vi "EventBuilder.publish event data service.vi"(0 "i ref in":refnum<vi>, 1 "eventID":i32=-1, 2 "eventData":T1, 3 "ms timeout (10000)":i32=10000, 5 "error in (no error)":errorcluster) -> (14 "i ref out":refnum<vi>, 17 "timed out":bool, 19 "error out":errorcluster)   [LabVIEW 2014, in "EventBuilder.lvlib"]
doc: "Publishes the service \"EVENTBUILDERNAME_eventData\".\n\nIf the service does not exist, it will be created. If the service data changes its size, the service is destroyed and recreated."
uses:
  EventBuilder.lvlib
  CS_Core/CSSystem/CoreDefs/CoreDefs.rawDataType.ctl
  CS_Core/CSSystem/CSSystemLib/CSSystemLib.lvlib
  CSlibraries-extern/DimLVEvent/LVDimInterface/LVDimInterface.lvlib
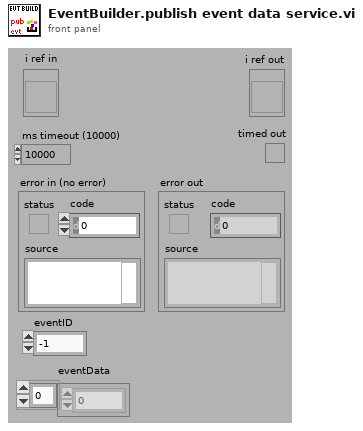
[diagram p1: front panel]
types:
  T1 = typedef "CoreDefs.rawDataType.ctl" = i8[]
  T2 = typedef "EventBuilder.lvlib/EventBuilder.i attribute.ctl" = cluster{"header":string, "DAQObjs":string[], "headerID":dbl, "eventID":i32, "dataDescriptionID":i32, "eventDataID":i32, "eventDataSize":i32, "dataDescriptionSize":i32}
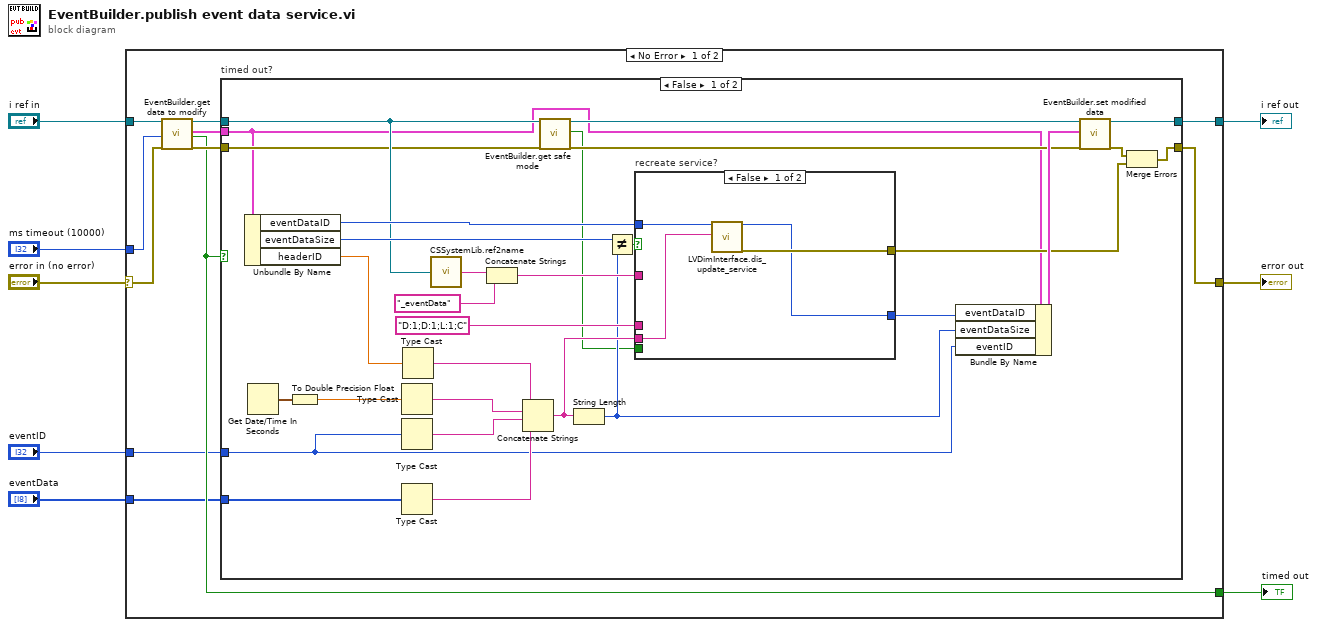
[diagram p0: block diagram]
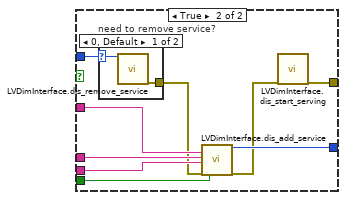
[diagram p2: hidden frame]
diagram:
  n1 = case shown="No Error" "error in (no error)" {
    selector: "error in (no error)" -> [w11 w67]
    tunnel: "i ref in" -> [w19 w68]
    tunnel: [w18 w67] -> w5
    tunnel: [w17 w68] -> w7
    tunnel: "ms timeout (10000)" -> [w13 _]
    tunnel: [w12 _] -> w3
    tunnel: "eventData" -> [w10 _]
    tunnel: "eventID" -> [w9 _]
    frame No Error {
      n2 = call "EventBuilder.get data to modify.vi"("i ref in"=w19, "ms timeout (10000)"=w13, "error in (no error)"=w11) -> ("i ref out"=w16:refnum<vi>, "i attribute"=w14:T2, "timed out"=w12:bool, "error out"=w15:errorcluster)  [unwired: 13 in]
      n3 = case "timed out?" shown="False" w12 {
        tunnel: [w39 w65] -> w18
        tunnel: [w49 w66] -> w17
        tunnel: w16 -> [w25 w66]
        tunnel: w15 -> [w23 w65]
        tunnel: w14 -> [w21 _]
        tunnel: w10 -> [w31 _]
        tunnel: w9 -> [w26 _]
        frame False {
          n4 = Unbundle By Name(w21) -> ("eventDataID"=w33:i32, "eventDataSize"=w35:i32, "headerID"=w30:dbl)
          n5 = Get Date/Time In Seconds() -> (seconds since 1Jan1904=w44:timestamp)
          n6 = To Double Precision Float(number=w44) -> (double precision float=w37:dbl)
          n7 = Type Cast(x=w37) -> (*(type *) &x=w43:string)  [unwired: 1 in]
          n8 = Type Cast(x=w26) -> (*(type *) &x=w28:string)  [unwired: 1 in]
          n9 = Type Cast(x=w31) -> (*(type *) &x=w27:string)  [unwired: 1 in]
          n10 = Type Cast(x=w30) -> (*(type *) &x=w29:string)  [unwired: 1 in]
          n11 = call "CSSystemLib.ref2name.vi"("obj refnum"=w25) -> ("name"=w48:string)
          n12 = Concatenate Strings(w48, "_eventData" ("string")) -> (w46:string)
          n13 = Concatenate Strings(w29, w43, w28, w27) -> (w36:string)
          n14 = call "EventBuilder.get safe mode.vi"("i ref in"=w25, "error in (no error)"=w23) -> ("i ref out"=w24:refnum<vi>, "safeMode"=w20:bool, "error out"=w22:errorcluster)  [unwired: 15 in]
          n15 = String Length(string=w36) -> (length=w32:i32)
          n16 = Not Equal?(x=w35, y=w32) -> (x != y?=w34:bool)
          n17 = case "recreate service?" shown="False" w34 {
            tunnel: w46 -> [_ w62]
            tunnel: "D:1;D:1;L:1;C" ("typeDescriptor") -> [_ w61]
            tunnel: [w51 w60] -> w42
            tunnel: [w52 w56] -> w38
            tunnel: w36 -> [w50 w59]
            tunnel: w33 -> [w53 w58]
            tunnel: w20 -> [_ w54]
            frame False {
              n18 = call "LVDimInterface.dis_update_service.vi"("my_serviceID"=w53, "data"=w50) -> ("my_serviceID out"=w51:i32, "error out"=w52:errorcluster)  [unwired: 15 in, 1 out]
            }
            frame True {
              n19 = case "need to remove service?" shown="0, Default" w58 {
                selector: w58 -> [w64 _]
                tunnel: [w63 _] -> w57
                frame 0, Default {
                  n20 = call "LVDimInterface.dis_remove_service.vi"("my_serviceID"=w64) -> ("error out"=w63:errorcluster)  [unwired: 18 in]
                }
                frame -1 {
                }
              }
              n21 = call "LVDimInterface.dis_add_service.vi"("serviceName"=w62, "typeDescriptor"=w61, "data"=w59, "error in (no error)"=w57, "safeMode"=w54) -> ("my_serviceID"=w60:i32, "error out"=w55:errorcluster)  [unwired: 13 in]
              n22 = call "LVDimInterface.dis_start_serving.vi"("error in (no error)"=w55) -> ("error out"=w56:errorcluster)  [unwired: 17 in, 1 out]
            }
          }
          n23 = Bundle By Name(cluster=w21, "eventDataID"=w42, "eventDataSize"=w32, "eventID"=w26) -> (w41:T2)
          n24 = call "EventBuilder.set modified data.vi"("i ref in"=w24, "i attribute"=w41, "error in (no error)"=w22) -> ("i ref out"=w49:refnum<vi>, "error out"=w40:errorcluster)  [unwired: 15 in]
          n25 = Merge Errors(w40, w38) -> (w39:errorcluster)
        }
        frame True {
        }
      }
    }
    frame Error {
    }
  }
  "error out" <- w5
  "i ref out" <- w7
  "timed out" <- w3
